vi "forceScreenshot.vi"   [LabVIEW 2013]
uses:
  System.ServiceModel
  G:/gitRepositories/TestProjects/WCFTest/WCFComputerLibrary/bin/Debug/WCFComputerLibrary.dll
  WCFComputerLibrary/bin/Debug/WCFComputerLibrary.dll
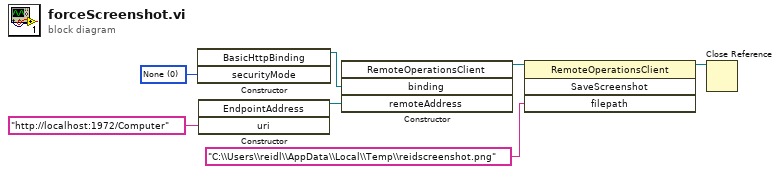
[diagram p0: block diagram]
diagram:
  w7 = 0 items=["None", "Transport", "Message", "TransportWithMessageCredential", "TransportCredentialOnly"] ("securityMode")
  n1 = constructor class="BasicHttpBinding"("securityMode"=w7) -> (reference out=w5:refnum<k24>)  [unwired: 3 in, 3 out]
  n2 = constructor class="EndpointAddress"("uri"="http://localhost:1972/Computer") -> (reference out=w4:refnum<k24>)  [unwired: 3 in, 3 out]
  n3 = constructor class="RemoteOperationsClient"("binding"=w5, "remoteAddress"=w4) -> (reference out=w3:refnum<k24>)  [unwired: 3 in, 4 out]
  n4 = invoke class="RemoteOperationsClient" method="SaveScreenshot"(reference=w3, "filepath"="C:\\Users\\reidl\\AppData\\Local\\Temp\\reidscreenshot.png") -> (reference out=w1:refnum<k24>)  [unwired: 2 in, 3 out]
  n5 = Close Reference(reference=w1) -> ()  [unwired: 1 in, 1 out]
